vi "fdyn_calc_xd.vi"(2 "data":variant, 3 "t":dbl, 4 "x":dbl[](array[numeric])) -> (0 "error out":errorcluster, 1 "dx/dt":dbl[](array[numeric]))   [LabVIEW 2017, in "NI_Kinematics.lvlib"]
uses:
  <vilib>/robotics/Kinematics/NI_Kinematics.lvlib
  <vilib>/robotics/Kinematics/dyn/fdyn_helper_data.ctl
  <vilib>/robotics/Kinematics/Robot/NI_Robotics_Serial Robot Arm.lvclass
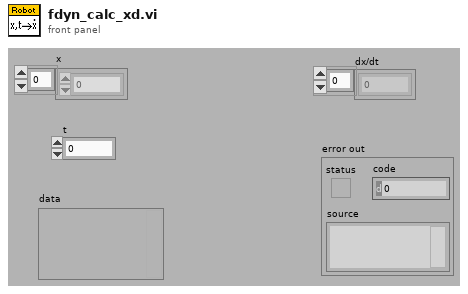
[diagram p1: front panel]
types:
  T1 = typedef "NI_Kinematics.lvlib/fdyn_helper_data.ctl" = cluster{"Robot In":refnum<class "NI_Robotics_Serial Robot Arm.lvclass">, "Torque Function":refnum<vi>, "Torque Function Data":variant}
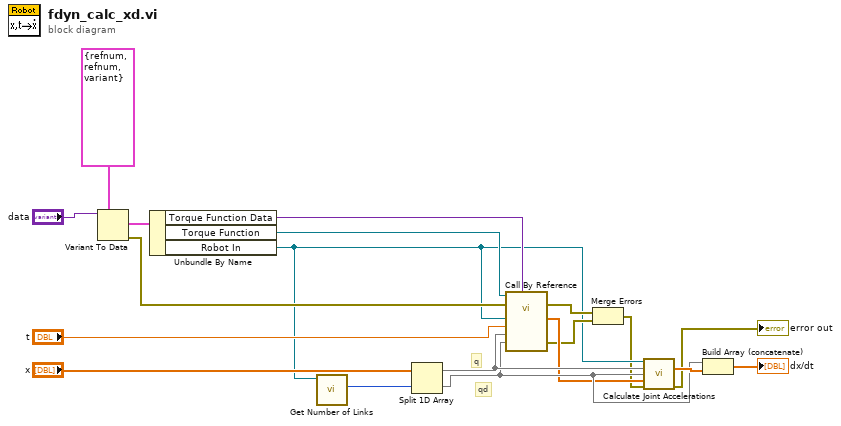
[diagram p0: block diagram]
diagram:
  # "qd"
  # "q"
  n1 = Variant To Data(type=T1 {"Robot In"=refnum, "Torque Function"=refnum, "Torque Function Data"=variant} ("fdyn_helper_data"), Variant="data") -> (data=w18:T1, error out=w4:errorcluster)  [unwired: 1 in]
  n2 = Unbundle By Name(w18) -> ("Torque Function Data"=w10:variant, "Torque Function"=w11:refnum<vi>, "Robot In"=w3:refnum<class "NI_Robotics_Serial Robot Arm.lvclass">)
  n3 = call <vilib>:"Get Number of Links.vi"("serial arm in"=w3) -> ("number of links"=w14:i32)  [unwired: 8 in, 2 out]
  n4 = Split 1D Array(array="x", index=w14) -> (first subarray=w8:dbl[], second subarray=w7:dbl[])
  n5 = call-by-ref "?"(reference=w11, error in=w4, "data"=w10, "qd"=w7, "q"=w8, "t"="t", "Robot.lvclass"=w3) -> (error out=w12:errorcluster, 0:"error out"=w5:errorcluster, "tau"=w6:dbl[])  [unwired: 5 in, 1 out]
  n6 = Merge Errors(w12, w5) -> (w2:errorcluster)
  n7 = call <vilib>:"Calculate Joint Accelerations.vi"("serial arm in"=w3, "joint positions"=w8, "joint velocities"=w7, "torques"=w6, "error in (no error)"=w2) -> ("joint accelerations"=w17:dbl[], "error out"=→"error out":errorcluster)  [unwired: 8 in, 1 out]
  n8 = Build Array (concatenate)(w7, w17) -> (→"dx/dt":dbl[])
